vi "FlexRefMemStimulusModel.vi"(11 "High Level":dbl=1.0) -> (3 "Out 1":dbl)   [LabVIEW 2010]
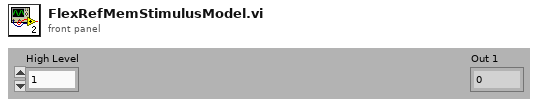
[diagram p1: front panel]
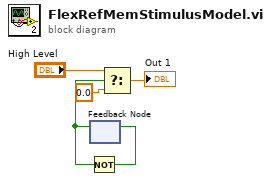
[diagram p0: block diagram]
diagram:
  n1 = feedback #1() -> (w2:bool)  [unwired: 1 in]
  n2 = Not(x=w2) -> (.not. x?=w1:bool)
  n3 = feedback-in #1(w1) -> ()
  n4 = Select(t="High Level", s=w2, f=0.0) -> (s? t:f=→"Out 1":dbl)
